vi "WriteParams.vi"(0 "CH1":dbl, 1 "CH5":dbl, 2 "CH6":dbl, 5 "CH2":dbl, 7 "CH3":dbl, 9 "CH4":dbl, 11 "error in (no error)":errorcluster, 12 "CH7":dbl, 13 "CH8":dbl) -> (15 "error out":errorcluster)   [LabVIEW 2014]
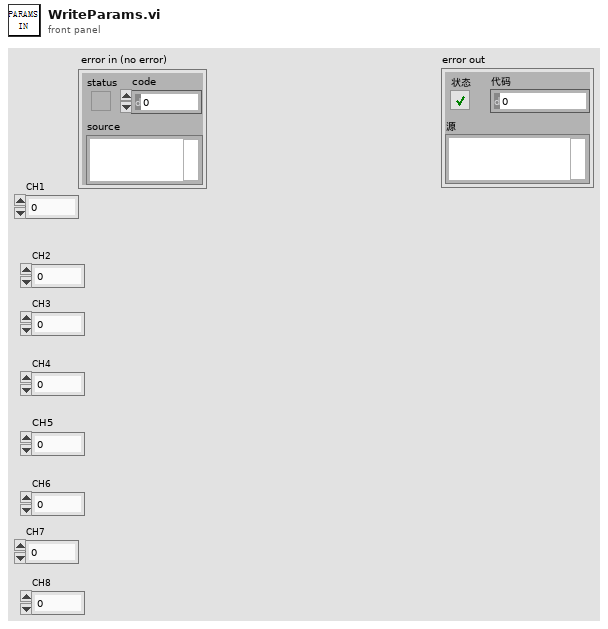
[diagram p1: front panel]
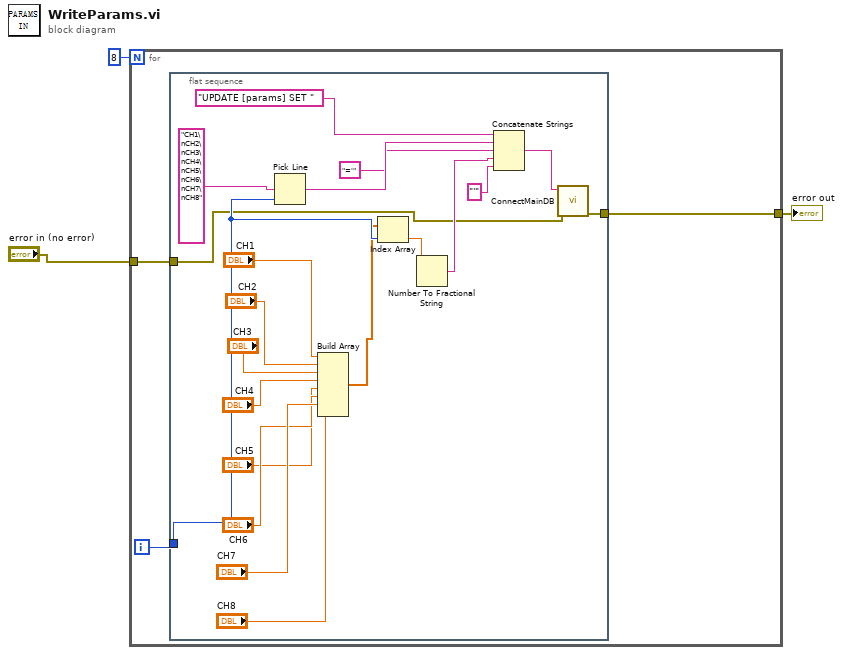
[diagram p0: block diagram]
diagram:
  n1 = for {
    N: 8 -> [_]
    tunnel: "error in (no error)" -> [w5]
    tunnel: [w4] -> w1
    i -> [w6]
    n2 = flat-sequence {
      tunnel: w6 -> [w23]
      tunnel: [w17] -> w4
      tunnel: w5 -> [w7]
      frame #0 {
        n3 = Pick Line(multi-line string="CH1\nCH2\nCH3\nCH4\nCH5\nCH6\nCH7\nCH8" ("多行字符串"), line index=w23) -> (output string=w24:string)  [unwired: 1 in]
        n4 = Build Array("CH1", "CH2", "CH3", "CH4", "CH5", "CH6", "CH7", "CH8") -> (w8:dbl[])
        n5 = Index Array(array=w8, index=w23) -> (element=w21:dbl)
        n6 = Number To Fractional String(number=w21) -> (F-format string=w20:string)  [unwired: 3 in]
        n7 = Concatenate Strings("UPDATE [params] SET ", w24, "='", w20, "'") -> (w18:string)
        n8 = call "ConnectMainDB.vi"("error in (no error)"=w7, "SQL query"=w18) -> ("error out"=w17:errorcluster)  [unwired: 8 in, 1 out]
      }
    }
  }
  "error out" <- w1
